vi "read.vi"(6 "call chain index (1)":i32=1, 7 "vi ref (caller)":refnum<vi>, 8 "error in (no error)":errorcluster) -> (0 "error out":errorcluster, 1 "plan sections":string[](array[string]), 2 "indices":i32[](array[numeric]), 3 "refnums":refnum<vi>[](array[refnum]), 4 "section settings":T1[][](array[typedef]), 5 "labels":string[](array[string]))   [LabVIEW 2024, in "controls manager.lvlib"]
uses:
  controls manager.lvlib
  key value pair.ctl
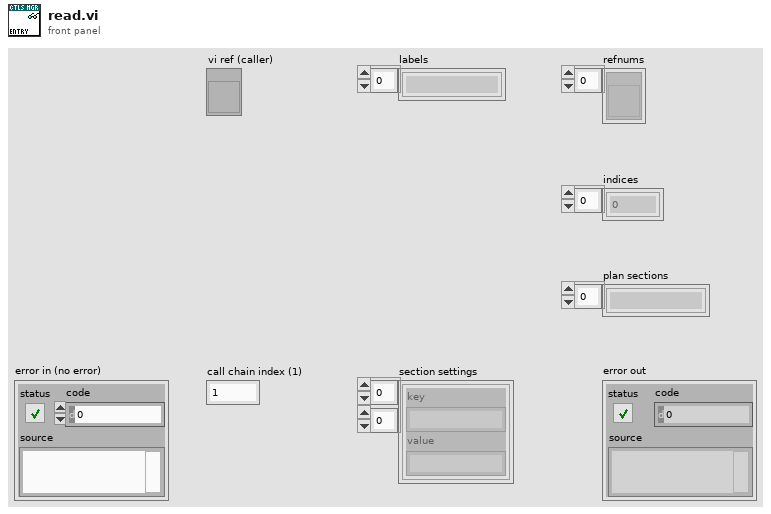
[diagram p1: front panel]
types:
  T1 = typedef "controls manager.lvlib/key value pair.ctl" = cluster{"key":string, "value":string}
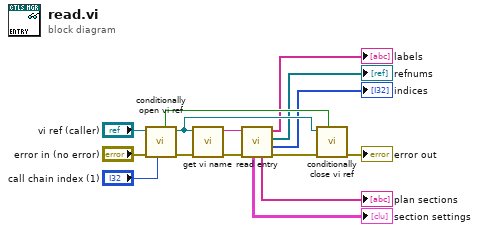
[diagram p0: block diagram]
diagram:
  n1 = call "conditionally open vi ref.vi"("call chain index (1)"="call chain index (1)", "error in (no error)"="error in (no error)", "vi ref in"="vi ref (caller)") -> ("error out"=w15:errorcluster, "vi ref out"=w12:refnum<vi>, "new ref?"=w11:bool)  [unwired: 6 in]
  n2 = call "get vi name.vi"("error in (no error)"=w15, "vi ref"=w12) -> ("error out"=w8:errorcluster, "vi name"=w6:string)  [unwired: 8 in]
  n3 = call "read entry.vi"("error in (no error)"=w8, "id"=w6) -> ("error out"=w7:errorcluster, "indices"=→"indices":i32[], "refnums"=→"refnums":refnum<vi>[], "labels"=→"labels":string[], "plan sections"=→"plan sections":string[], "section settings"=→"section settings":T1[][])  [unwired: 4 in]
  n4 = call "conditionally close vi ref.vi"("new ref?"=w11, "error in (no error)"=w7, "vi ref"=w12) -> ("error out"=→"error out":errorcluster)  [unwired: 8 in]
